vi "Table_MergePreviousConfiguration.vi"(8 "error in (no error)":errorcluster, 10 "Selections":string[][](array[string]), 11 "Path":path) -> (0 "error out":errorcluster, 2 "Data":string[](array[string]), 3 "Path Out":path)   [LabVIEW 2012, in "TableSupportLib.lvlib"]
uses:
  TableSupportLib.lvlib
  Table_LimitSettings.ctl
  Table_Globals.vi
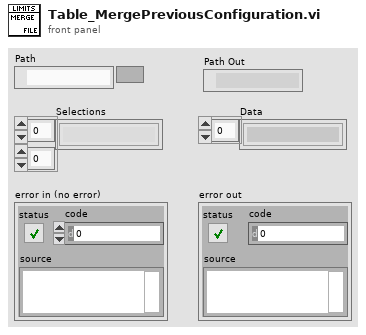
[diagram p1: front panel]
types:
  T1 = typedef "TableSupportLib.lvlib/Table_LimitSettings.ctl" = cluster{"High":dbl, "High Warning":dbl, "Low Warning":dbl, "Low":dbl}
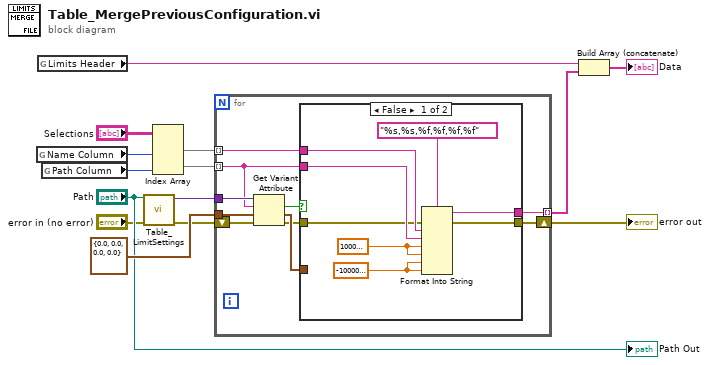
[diagram p0: block diagram]
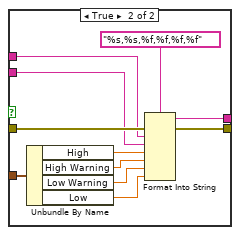
[diagram p2: hidden frame]
diagram:
  n1 = global read "Table_Globals.vi" "Name Column"() -> (w9:i32)
  n2 = global read "Table_Globals.vi" "Limits Header"() -> (w13:string)
  n3 = global read "Table_Globals.vi" "Path Column"() -> (w8:i32)
  n4 = call "Table_LimitSettings.vi"("error in"="error in (no error)", "file path (use dialog)"="Path") -> ("error out"=w4:errorcluster, "Limit Settings"=w5:variant)  [unwired: 8 in]
  n5 = Index Array(array="Selections", index (col) #1=w9, index (col) #2=w8) -> (element #1=w6:string[], element #2=w10:string[])  [unwired: 2 in]
  n6 = for {
    shift-right: [w16] -> w11
    shift-left: w4 -> [w24]
    tunnel: w5 -> [w23]
    tunnel: w6 -> [w19] mode=indexing
    tunnel: T1 {"High"=0.0, "High Warning"=0.0, "Low Warning"=0.0, "Low"=0.0} -> [w22]
    tunnel: w10 -> [w18] mode=indexing
    tunnel: [w15] -> w12 mode=indexing
    n7 = Get Variant Attribute(Variant=w23, name=w18, default value (empty Variant)=w22, error in=w24) -> (found=w20:bool, value=w21:T1, error out=w17:errorcluster)  [unwired: 1 out]
    n8 = case shown="False" w20 {
      tunnel: w21 -> [_ w43]
      tunnel: w19 -> [w31 w34]
      tunnel: w18 -> [w30 w39]
      tunnel: w17 -> [w29 w41]
      tunnel: [w28 w40] -> w16
      tunnel: [w27 w33] -> w15
      frame False {
        w26 = -10000000000.0
        w25 = 10000000000.0
        n9 = Format Into String(format string="%s,%s,%f,%f,%f,%f", error in=w29, w31, w30, w25, w25, w26, w26) -> (resulting string=w27:string, error out=w28:errorcluster)  [unwired: 1 in]
      }
      frame True {
        n10 = Unbundle By Name(w43) -> ("High"=w38:dbl, "High Warning"=w37:dbl, "Low Warning"=w36:dbl, "Low"=w35:dbl)
        n11 = Format Into String(format string="%s,%s,%f,%f,%f,%f", error in=w41, w34, w39, w38, w37, w36, w35) -> (resulting string=w33:string, error out=w40:errorcluster)  [unwired: 1 in]
      }
    }
  }
  "error out" <- w11
  n12 = Build Array (concatenate)(w13, w12) -> (→"Data":string[])
  "Path Out" <- "Path"
